vi "Close.vi"(8 "error in":errorcluster, 11 "DBC Communication in":refnum<class "DBC Communication.lvclass">) -> (0 "error out":errorcluster, 3 "DBC Communication out":refnum<class "DBC Communication.lvclass">)   [LabVIEW 2024, in "DBC Communication.lvclass"]
uses:
  DBC Communication.lvclass
  DBC Communication.lvclass/DBC Communication.ctl
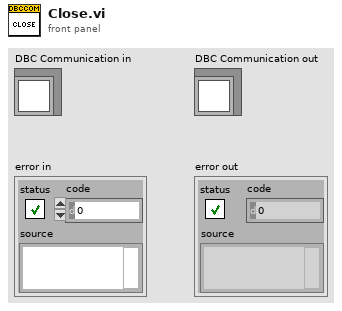
[diagram p1: front panel]
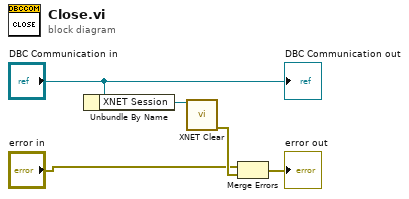
[diagram p0: block diagram]
diagram:
  n1 = Unbundle By Name("DBC Communication in") -> ("XNET Session"=w4:refnum<k21>)
  n2 = call <vilib>:"XNET Clear.vi"("session in"=w4) -> ("error out"=w3:errorcluster)  [unwired: 14 in]
  n3 = Merge Errors("error in", w3) -> (→"error out":errorcluster)
  "DBC Communication out" <- "DBC Communication in"
